vi "System Message.vi"(7 "Sys. Msg. Source":T1, 8 "error in":errorcluster, 9 "Payload":variant, 10 "Identifier":string) -> (0 "error out":errorcluster)   [LabVIEW 2022 SP3, in "Settings.lvlib"]
doc: "_____\nCreated using DQMH Event Scripter 7.0.0.1280."
uses:
  Settings.lvlib
  Libraries/hse-libraries/Source/hse-dqmh/Controls/System Message Source.ctl
  System Message Argument--cluster.ctl
  Libraries/hse-libraries/Source/hse-dqmh/hse-dqmh.lvlib
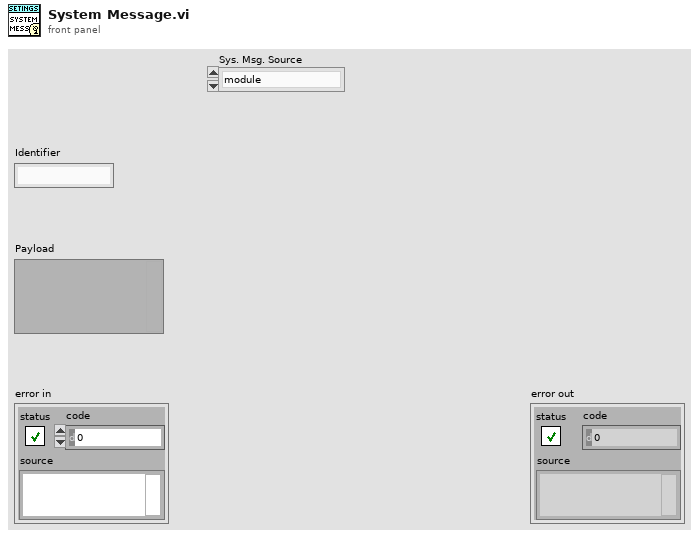
[diagram p1: front panel]
types:
  T1 = typedef "hse-dqmh.lvlib/System Message Source.ctl" = enum16{"module", "application", "network"}
  T2 = typedef "Settings.lvlib/System Message Argument--cluster.ctl" = cluster{"Identifier":string, "Payload":variant, "Sys. Msg. Source":T1, "Sys. Msg. Origin":string}
  T3 = typedef "Settings.lvlib/Broadcast Events--cluster.ctl" = cluster{"Module Did Init":refnum<user-event>, "Status Updated":refnum<user-event>, "Error Reported":refnum<user-event>, "Did Something":refnum<user-event>, "Module Did Stop":refnum<user-event>, "Update Module Execution Status":refnum<user-event>, "System Message":refnum<user-event>}
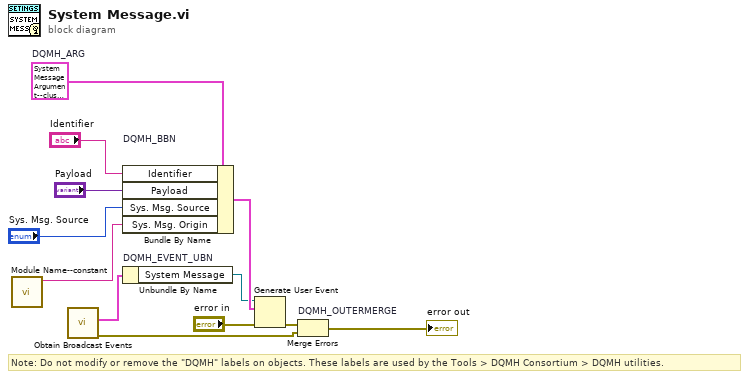
[diagram p0: block diagram]
diagram:
  w7 = T2 {"Identifier"="", "Payload"=variant, "Sys. Msg. Source"=enum."module", "Sys. Msg. Origin"=""}  # DQMH_ARG
  # "Note: Do not modify or remove the \"DQMH\" labels on objects. These labels are used by the Tools > DQMH Consortium > DQMH utilities."
  n1 = call "Module Name--constant.vi"() -> ("Module Name"=w3:string)  [unwired: 11 in]
  n2 = call "Obtain Broadcast Events.vi"() -> ("error out"=w2:errorcluster, "Settings Broadcast Events"=w1:T3)  [unwired: 10 in]
  n3 = Bundle By Name "DQMH_BBN"(cluster=w7, "Identifier"="Identifier", "Payload"="Payload", "Sys. Msg. Source"="Sys. Msg. Source", "Sys. Msg. Origin"=w3) -> (w10:T2)
  n4 = Unbundle By Name "DQMH_EVENT_UBN"(w1) -> ("System Message"=w9:refnum<user-event>)
  n5 = Generate User Event(user event=w9, event data cluster=w10, error in="error in") -> (error out=w8:errorcluster)  [unwired: 1 in, 1 out]
  n6 = Merge Errors "DQMH_OUTERMERGE"(w8, w2) -> (→"error out":errorcluster)
